vi "updateTestResult.vi"(8 "error in (no error)":errorcluster, 9 "TestResult":T1, 10 "TaskName":string, 11 "TestLstRef in":refnum<vi>) -> (0 "error out":errorcluster, 3 "TestLstRef out":refnum<vi>)   [LabVIEW 2010, in "pdbm_test_system.lvlib"]
uses:
  pdbm_test_system.lvlib
  pdbm_tasks/UsrDefine/TestResult.ctl
  pdbm_tasks/pdbm_tasks.lvlib
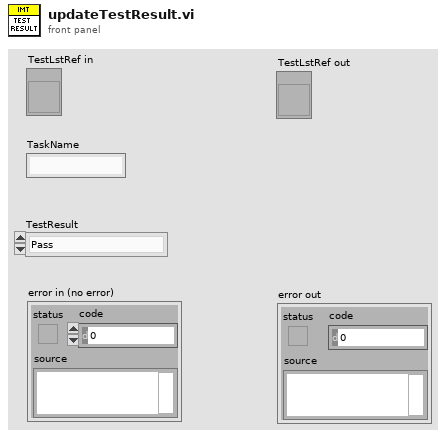
[diagram p1: front panel]
types:
  T1 = typedef "pdbm_tasks.lvlib/TestResult.ctl" = enum16{"Pass", "Fail", "Warning"}
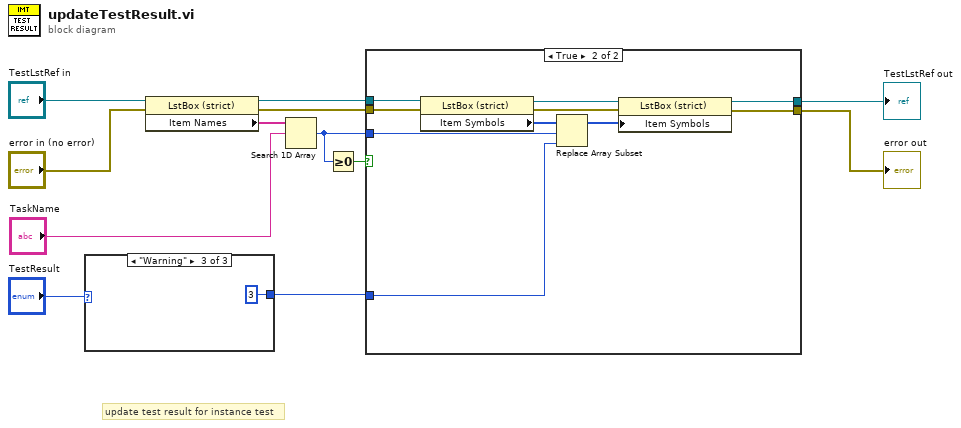
[diagram p0: block diagram]
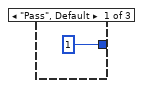
[diagram p2: hidden frame]
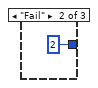
[diagram p3: hidden frame]
diagram:
  # "update test result for instance test"
  n1 = case shown="\"Warning\"" "TestResult" {
    tunnel: [1 2 3] -> w1
    frame "Pass", Default {
    }
    frame "Fail" {
    }
    frame "Warning" {
    }
  }
  n2 = property class="LstBox (strict)"(reference="TestLstRef in", error in="error in (no error)") -> (reference out=w11:refnum<vi>, error out=w10:errorcluster, "Item Names"=w12:string[])
  n3 = Search 1D Array(1D array=w12, element="TaskName") -> (index of element=w8:i32)  [unwired: 1 in]
  n4 = Greater Or Equal To 0?(x=w8) -> (x >= 0?=w9:bool)
  n5 = case shown="True" w9 {
    tunnel: w11 -> [w17 w27]
    tunnel: w10 -> [w16 w26]
    tunnel: w1 -> [_ w24]
    tunnel: w8 -> [_ w23]
    tunnel: [w17 w19] -> w4
    tunnel: [w16 w18] -> w3
    frame False {
    }
    frame True {
      n6 = property class="LstBox (strict)"(reference=w27, error in=w26) -> (reference out=w22:refnum<vi>, error out=w21:errorcluster, "Item Symbols"=w25:i32[])
      n7 = Replace Array Subset(array=w25, new element=w24, index=w23) -> (w20:i32[])
      n8 = property class="LstBox (strict)"(reference=w22, error in=w21, "Item Symbols"=w20) -> (reference out=w19:refnum<vi>, error out=w18:errorcluster)
    }
  }
  "TestLstRef out" <- w4
  "error out" <- w3
